vi "ILC_servo_sim.vi"() -> ()   [LabVIEW 2021]
uses:
  <vilib>/addons/Control Design/_Model Construction/Model Creation.llb/Model Creation SubVI/cd_Create Transfer Function Model.vi
  <vilib>/addons/Control Design/_Model Construction/Model Information.llb/Model Information SubVIs/cd_Set Names To TF Model.vi
  <vilib>/addons/Control Design/_Utility/Model Viewer.llb/Model Viewer SubVI/cd_Draw Transfer Function Equation (TF).vi
  <vilib>/addons/Control Design/_Model Conversions/Continuous and Discrete.llb/Continuous and Discrete SubVI/cd_Convert Continuous to Discrete (TF).vi
  <vilib>/addons/Control Design/_Model Conversions/Model Type.llb/Model Conversion SubVI/cd_Convert Transfer Function to State-Space Model.vi
  <vilib>/addons/Control Design/_Model Construction/Model Information.llb/Model Information SubVIs/cd_Get Matrices From SS Model.vi
  <vilib>/imath/engines/lvmath2/RunTimeEngine/RangeToken/NIMS_Range_R2 - Integer.vi
  <instcachedir>/0/NIMS_Range_R2 - Integer_5BFA5D3E872644D4A9D01FD9E43E5B44.lvgen/NIMS_Range_R2 - Integer_5BFA5D3E872644D4A9D01FD9E43E5B44_000.vi
  <vilib>/imath/engines/lvmath2/RunTimeEngine/CommandStatement/MC_CommandStatement_break.vi
  <vilib>/imath/engines/lvmath2/RunTimeEngine/ArithmeticOperatorToken/NIMS_ArithmeticOperator_powermx(M,M).vi
  <vilib>/imath/engines/lvmath2/RunTimeEngine/ArithmeticOperatorToken/NIMS_ArithmeticOperator_multmx.vi
  <instcachedir>/0/NIMS_ArithmeticOperator_multmx_E4383E337866406DBBEFAB93A2F250EA.lvgen/NIMS_ArithmeticOperator_multmx_E4383E337866406DBBEFAB93A2F250EA_007.vi
  <instcachedir>/0/NIMS_ArithmeticOperator_multmx_E4383E337866406DBBEFAB93A2F250EA.lvgen/NIMS_ArithmeticOperator_multmx_E4383E337866406DBBEFAB93A2F250EA_008.vi
  <vilib>/imath/engines/lvmath2/RunTimeEngine/IndexReplace/NIMS M(S,S)=M.vi
  <instcachedir>/0/NIMS M(S,S)=M_22574F0A0D8E490084047103BBBC33E2.lvgen/NIMS M(S,S)=M_22574F0A0D8E490084047103BBBC33E2_000.vi
  <vilib>/imathl/engines/lvmath/Functions/Error Handling/Create Error.vi
  <vilib>/imath/engines/lvmath2/RunTimeEngine/ErrorHandling/NIMS_Create Error From Enums.vi
  <vilib>/imath/engines/lvmath2/RunTimeEngine/RangeToken/NIMS_Range.vi
  <instcachedir>/0/NIMS_Range_55C28A69746948C3BE8F3B076E0CF496.lvgen/NIMS_Range_55C28A69746948C3BE8F3B076E0CF496_001.vi
  <vilib>/imath/engines/lvmath2/RunTimeEngine/IndexReplace/NIMS M(S,S)=S.vi
  <instcachedir>/0/NIMS M(S,S)=S_7FF91F16E3664466856A44581A7FF6F9.lvgen/NIMS M(S,S)=S_7FF91F16E3664466856A44581A7FF6F9_002.vi
  <vilib>/imath/engines/lvmath2/RunTimeEngine/NodeEndStatement/NIMS_NodeEndStatement_Output.vi
  <instcachedir>/0/NIMS_NodeEndStatement_Output_53EC0D466D134D7ABD903AC30B43404B.lvgen/NIMS_NodeEndStatement_Output_53EC0D466D134D7ABD903AC30B43404B_010.vi
  <instcachedir>/0/NIMS_NodeEndStatement_Output_53EC0D466D134D7ABD903AC30B43404B.lvgen/NIMS_NodeEndStatement_Output_53EC0D466D134D7ABD903AC30B43404B_009.vi
  <instcachedir>/0/NIMS_NodeEndStatement_Output_53EC0D466D134D7ABD903AC30B43404B.lvgen/NIMS_NodeEndStatement_Output_53EC0D466D134D7ABD903AC30B43404B_003.vi
  <vilib>/imath/engines/lvmath2/RunTimeEngine/ErrorHandling/NIMS_Finalize Error.vi
  <vilib>/imath/engines/lvmath2/RunTimeEngine/BuiltInFunctions/zeros/NIMS_M=zeros(I32,I32).vi
  <vilib>/imath/engines/lvmath2/RunTimeEngine/IndexRead/NIMS M($,S).vi
  <instcachedir>/0/NIMS M($,S)_3E5749BBB62E49528D4765A77F1F6D98.lvgen/NIMS M($,S)_3E5749BBB62E49528D4765A77F1F6D98_002.vi
  <instcachedir>/0/NIMS M($,S)_3E5749BBB62E49528D4765A77F1F6D98.lvgen/NIMS M($,S)_3E5749BBB62E49528D4765A77F1F6D98_001.vi
  <vilib>/imath/engines/lvmath2/RunTimeEngine/ArithmeticOperatorToken/NIMS_ArithmeticOperator_multmx(M,CV).vi
  <instcachedir>/0/NIMS_ArithmeticOperator_multmx(M,CV)_A56766D51B5B40F3835DE1AFAAC1F0FE.lvgen/NIMS_ArithmeticOperator_multmx(M,CV)_A56766D51B5B40F3835DE1AFAAC1F0FE_002.vi
  <vilib>/imath/engines/lvmath2/RunTimeEngine/ArithmeticOperatorToken/NIMS_ArithmeticOperator_minus.vi
  <instcachedir>/0/NIMS_ArithmeticOperator_minus_686F2F9BA8D64789BA308312BA2E7296.lvgen/NIMS_ArithmeticOperator_minus_686F2F9BA8D64789BA308312BA2E7296_009.vi
  <vilib>/imath/engines/lvmath2/RunTimeEngine/IndexReplace/NIMS M($,S)=M.vi
  <instcachedir>/0/NIMS M($,S)=M_43283F335BC846D6ACA97A7D70262FEC.lvgen/NIMS M($,S)=M_43283F335BC846D6ACA97A7D70262FEC_001.vi
  <instcachedir>/0/NIMS_ArithmeticOperator_multmx_E4383E337866406DBBEFAB93A2F250EA.lvgen/NIMS_ArithmeticOperator_multmx_E4383E337866406DBBEFAB93A2F250EA_003.vi
  <vilib>/imath/engines/lvmath2/RunTimeEngine/BuiltInFunctions/norm/NIMS_norm(GM,DBL).vi
  <instcachedir>/0/NIMS_norm(GM,DBL)_D882E09FC0924E0F98CF38CBB78F43B9.lvgen/NIMS_norm(GM,DBL)_D882E09FC0924E0F98CF38CBB78F43B9_001.vi
  <vilib>/imath/engines/lvmath2/RunTimeEngine/IndexReplace/NIMS V(S)=S.vi
  <instcachedir>/0/NIMS V(S)=S_F56214BC46A343A9BE2E221E47313A2C.lvgen/NIMS V(S)=S_F56214BC46A343A9BE2E221E47313A2C_000.vi
  <vilib>/imath/engines/lvmath2/RunTimeEngine/IndexRead/NIMS V(S).vi
  <instcachedir>/0/NIMS V(S)_0488751826AF41519A22953C041130DC.lvgen/NIMS V(S)_0488751826AF41519A22953C041130DC_000.vi
  <vilib>/imath/engines/lvmath2/RunTimeEngine/ArithmeticOperatorToken/NIMS_ArithmeticOperator_plus.vi
  <instcachedir>/0/NIMS_ArithmeticOperator_plus_8086907561C54B16AC97E832CC9361D4.lvgen/NIMS_ArithmeticOperator_plus_8086907561C54B16AC97E832CC9361D4_002.vi
  <vilib>/imath/engines/lvmath2/RunTimeEngine/BuiltInFunctions/norm/NIMS_norm(GV,DBL).vi
  <instcachedir>/0/NIMS_norm(GV,DBL)_1596802B12A0462FBB989076B815DB12.lvgen/NIMS_norm(GV,DBL)_1596802B12A0462FBB989076B815DB12_001.vi
  <vilib>/imath/engines/lvmath2/RunTimeEngine/IndexReplace/NIMS M(S)=S.vi
  <instcachedir>/0/NIMS M(S)=S_C3A84BCB962A472CA66328840121DCD5.lvgen/NIMS M(S)=S_C3A84BCB962A472CA66328840121DCD5_001.vi
  <vilib>/imath/engines/lvmath2/RunTimeEngine/BuiltInFunctions/figure/NIMS_figure(I32).vi
  <vilib>/imath/engines/lvmath2/RunTimeEngine/BuiltInFunctions/plot/NIMS_plot(RM, RM, Str).vi
  <vilib>/addons/Control Design/_Model Conversions/NI_CD_Model Type.lvlib
  <vilib>/addons/Control Design/_Model Construction/NI_LinSys_Model Information.lvlib
  <vilib>/addons/Control Design/_Model Construction/NI_LinSys_Model Creation.lvlib
  <vilib>/addons/Control Design/_Utility/NI_CD_Model Viewer.lvlib
  <vilib>/addons/Control Design/_Model Conversions/NI_CD_Continuous and Discrete.lvlib
panel:
  in  "Polynomial Order":bool=TRUE
  in  "Sampling Time (s)":dbl format="%#.6p"
  in  "Model Name":string="G"
  out "Resulting Model":picture
  in  "Numerator":dbl[](array[numeric])=[1.0] format="%#.5g"
  in  "Denominator":dbl[](array[numeric])=[1.0, 2.0] format="%#.5g"
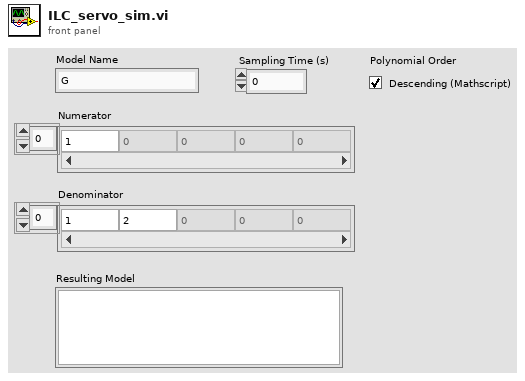
[diagram p1: front panel]
types:
  T1 = typedef "NI_LinSys_Model Typedefs.lvlib/CD Transfer Function Model (MIMO).ctl" = cluster{"properties":T2, "transfer function(s)":T3[][]}
  T2 = typedef "NI_LinSys_Model Typedefs.lvlib/CD General Elements.ctl" = cluster{"Model name":string, "Input names":string[], "Output names":string[], "Input Delays":dbl[], "Output Delays":dbl[], "Sampling Time":dbl, "Notes":string}
  T3 = typedef "NI_LinSys_Model Typedefs.lvlib/CD Transfer Function Model (SISO).ctl" = cluster{"Numerator":dbl[], "Denominator":dbl[], "delay":dbl}
  T4 = typedef "NI_LinSys_Model Typedefs.lvlib/CD State Space Model (MIMO).ctl" = cluster{"properties":T2, "A":dbl[][], "B":dbl[][], "C":dbl[][], "D":dbl[][], "StateNames":string[], "Transport Delay":dbl[][]}
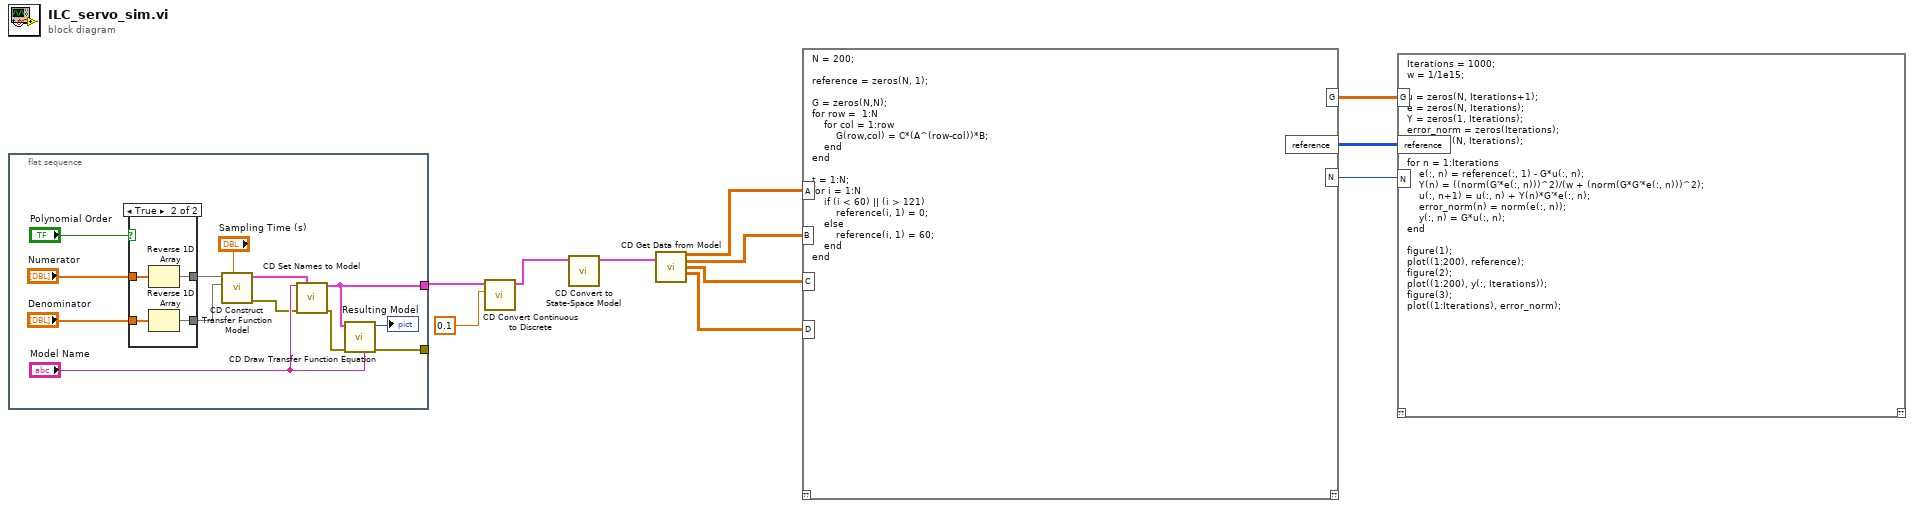
[diagram p0: block diagram]
diagram:
  n1 = flat-sequence {
    tunnel: [w18] -> w10
    tunnel: [w14] -> _
    frame #0 {
      n2 = case shown="True" "Polynomial Order" {
        tunnel: "Numerator" -> [w26 w30]
        tunnel: [w26 w29] -> w16
        tunnel: "Denominator" -> [w25 w28]
        tunnel: [w25 w27] -> w15
        frame False {
        }
        frame True {
          n3 = Reverse 1D Array(array=w30) -> (reversed array=w29:dbl[])
          n4 = Reverse 1D Array(array=w28) -> (reversed array=w27:dbl[])
        }
      }
      n5 = call-poly <vilib>:"CD Construct Transfer Function Model.vi"("Sampling Time (s)"="Sampling Time (s)", "Denominator"=w15, "Numerator"=w16) -> ("error out"=w12:errorcluster, "Transfer Function Model"=w17:T1)  [unwired: 7 in]
      n6 = call-poly <vilib>:"CD Set Names to Model.vi"("Model Name"="Model Name", "Transfer Function Model In"=w17, "error in (no error)"=w12) -> ("Model Out"=w18:T1, "error out"=w13:errorcluster)  [unwired: 11 in]
      n7 = call-poly <vilib>:"CD Draw Transfer Function Equation.vi"("Function Name (empty)"="Model Name", "error in (no error)"=w13, "Transfer Function Model"=w18) -> ("error out"=w14:errorcluster, "Equation"=→"Resulting Model":picture)  [unwired: 6 in, 1 out]
    }
  }
  n8 = call-poly <vilib>:"CD Convert Continuous to Discrete.vi"("Sampling Time (s)"=0.1, "Continuous Transfer Function Model"=w10) -> ("Discrete Transfer Function Model"=w9:T1)  [unwired: 8 in, 1 out]
  n9 = call-poly <vilib>:"CD Convert to State-Space Model.vi"("Transfer Function Model"=w9) -> ("State-Space Model"=w11:T4)  [unwired: 9 in, 1 out]
  n10 = call-poly <vilib>:"CD Get Data from Model.vi"("State-Space Model"=w11) -> ("Matrix A"=w4:dbl[][], "Matrix B"=w3:dbl[][], "Matrix C"=w2:dbl[][], "Matrix D"=w1:dbl[][])  [unwired: 10 in, 1 out]
  n11 = mathscript code="N = 200;\n\nreference = zeros(N, 1);\n\nG = zeros(N,N);\nfor row =  1:N \n    for col = 1:row\n        G(row,col) = C*(A^(row-col))*B;\n    end \nend\n\nt = 1:N;\nfor i = 1:N\n    if (i < 60) || (i > 121)\n        reference(i, 1) = 0;\n    else\n        reference(i, 1) = 60;\n    end\nend"("A"=w4, "B"=w3, "C"=w2, "D"=w1) -> ("G"=w6:cdb[][], "reference"=w7:i32[][], "N"=w5:i32)  [unwired: 1 in, 1 out]
  n12 = mathscript code="Iterations = 1000;\nw = 1/1e15;\n\nu = zeros(N, Iterations+1);\ne = zeros(N, Iterations);\nY = zeros(1, Iterations);\nerror_norm = zeros(Iterations);\ny = zeros(N, Iterations);\n\nfor n = 1:Iterations\n    e(:, n) = reference(:, 1) - G*u(:, n);\n    Y(n) = ((norm(G'*e(:, n)))^2)/(w + (norm(G*G'*e(:, n)))^2);\n    u(:, n+1) = u(:, n) + Y(n)*G'*e(:, n);\n    error_norm(n) = norm(e(:, n));\n    y(:, n) = G*u(:, n);\nend\n\nfigure(1);\nplot((1:200), reference);\nfigure(2);\nplot((1:200), y(:, Iterations));\nfigure(3);\nplot((1:Iterations), error_norm);"("G"=w6, "reference"=w7, "N"=w5) -> ()  [unwired: 1 in, 1 out]
